vi "Get VI Name From Reference.vi"(8 "error in (no error)":errorcluster, 11 "VI Ref":refnum<vi>) -> (0 "error out":errorcluster, 3 "VI Name":string)   [LabVIEW 2011]
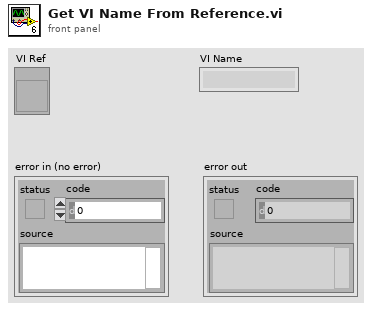
[diagram p1: front panel]
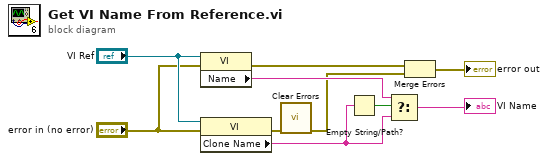
[diagram p0: block diagram]
diagram:
  n1 = property class="VI"(reference="VI Ref", error in="error in (no error)") -> (error out=w3:errorcluster, "Name"=w6:string)  [unwired: 1 out]
  n2 = property class="VI"(reference="VI Ref", error in="error in (no error)") -> (error out=w8:errorcluster, "Clone Name"=w7:string)  [unwired: 1 out]
  n3 = call <vilib>:"Clear Errors.vi"("error in (no error)"=w8) -> ("error out"=w1:errorcluster)  [unwired: 6 in]
  n4 = Empty String/Path?(string/path=w7) -> (empty?=w5:bool)
  n5 = Select(t=w6, s=w5, f=w7) -> (s? t:f=→"VI Name":string)
  n6 = Merge Errors(w3, w1) -> (→"error out":errorcluster)
